vi "PH_PP_CurrentMeas_Stop.vi"(0 "connection ID in":refnum<k5>, 5 "error in (no error)":errorcluster) -> (14 "No Data achieved due to Task Failure":bool, 15 "Error unpacking Data?":bool, 16 "Measurement Data":waveform(dbl)[](graph), 17 "Receveived Data Sets":T1[](array[typedef]), 18 "No Data achieved due to no Trigger Signal":bool, 19 "error out":errorcluster)   [LabVIEW 2014, in "PH_PP_CurrentMeas.lvlib"]
uses:
  PH_PP_CurrentMeas.lvlib
  PH_PP_CurrentMeas.Command.ctl
  PH_PP_CurrentMeas.CommandCluster.ctl
panel:
  in  "Dummy":T1
  in  "Command":T2=enum."CloseConnection"
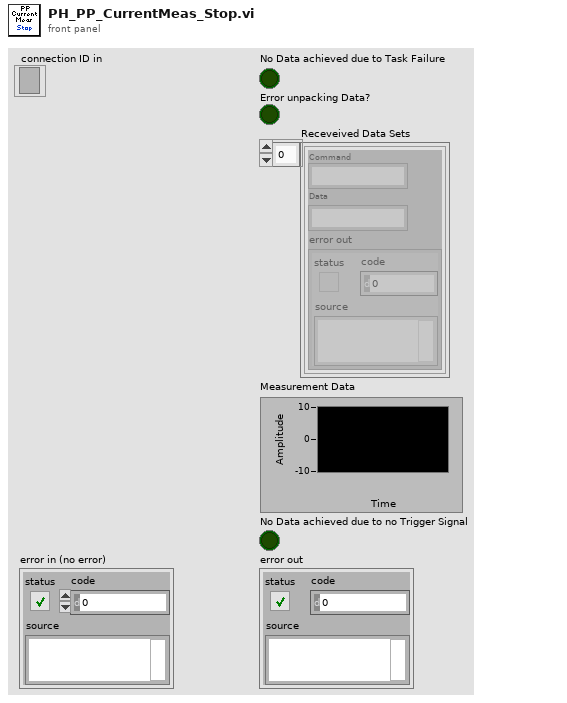
[diagram p1: front panel]
types:
  T1 = typedef "PH_PP_CurrentMeas.lvlib/PH_PP_CurrentMeas.CommandCluster.ctl" = cluster{"Command":string, "Data":string, "error out":errorcluster}
  T2 = typedef "PH_PP_CurrentMeas.lvlib/PH_PP_CurrentMeas.Command.ctl" = enum16{"StartDAQ", "StopDAQ", "GetDAQStatus", "CloseConnection"}
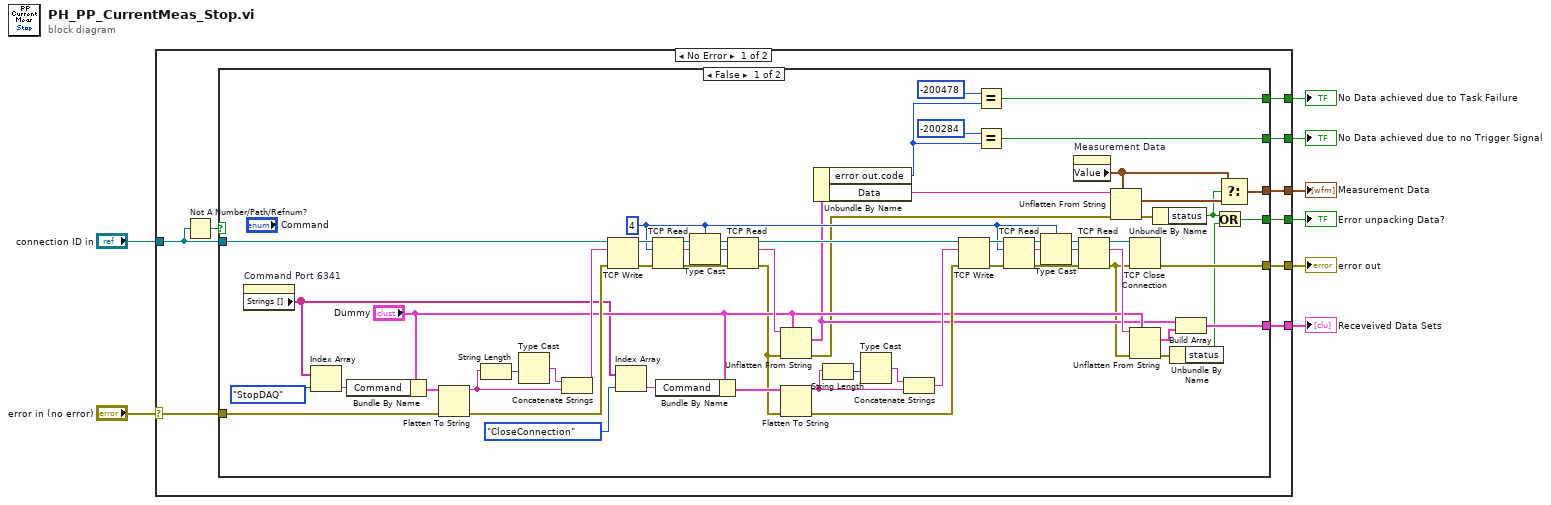
[diagram p0: block diagram]
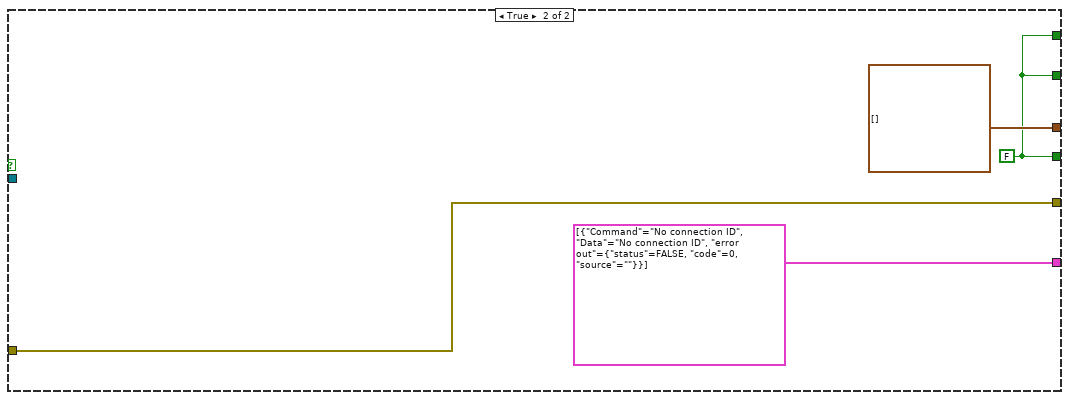
[diagram p2: hidden frame]
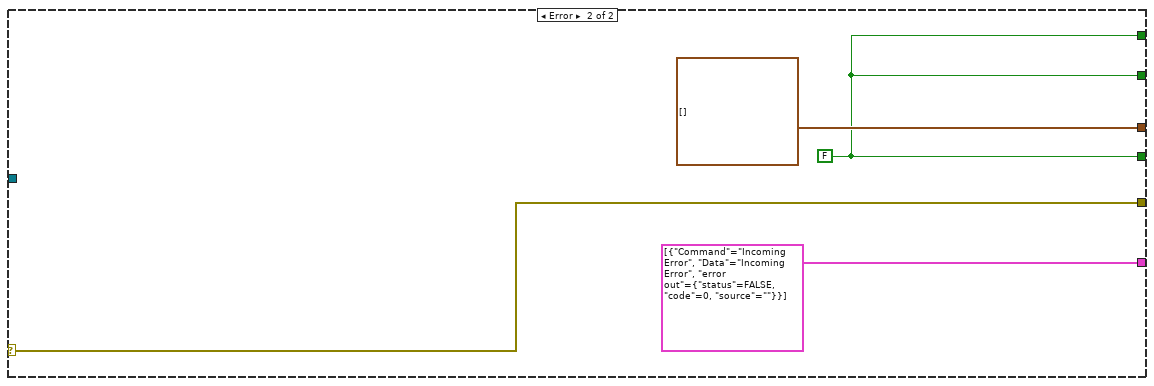
[diagram p3: hidden frame]
diagram:
  n1 = case shown="No Error" "error in (no error)" {
    selector: "error in (no error)" -> [w11 w83]
    tunnel: [w17 waveform(dbl)[] [] ("Value")] -> w8
    tunnel: "connection ID in" -> [w16 _]
    tunnel: [w15 w83] -> w6
    tunnel: [w14 T1[] [{"Command"="Incoming Error", "Data"="Incoming Error", "error out"={"status"=FALSE, "code"=0, "source"=""}}]] -> w5
    tunnel: [w12 w80] -> w4
    tunnel: [w10 w80] -> w2
    tunnel: [w9 w80] -> w1
    frame No Error {
      n2 = Not A Number/Path/Refnum?(number/path/refnum=w16) -> (NaN/Path/Refnum?=w13:bool)
      n3 = case shown="False" w13 {
        tunnel: [w57 waveform(dbl)[] [] ("Value")] -> w17
        tunnel: w11 -> [w56 w79]
        tunnel: w16 -> [w55 _]
        tunnel: [w54 w79] -> w15
        tunnel: [w32 T1[] [{"Command"="No connection ID", "Data"="No connection ID", "error out"={"status"=FALSE, "code"=0, "source"=""}}]] -> w14
        tunnel: [w24 w76] -> w12
        tunnel: [w21 w76] -> w10
        tunnel: [w18 w76] -> w9
        frame False {
          w34 = 4 ("bytes to read")
          n4 = property on="Command Port 6341" class="Enum (strict)"() -> ("Strings []"=w37:string[])  [unwired: 2 in, 2 out]
          n5 = Index Array(array=w37, index=PH_PP_CurrentMeas.Command."StopDAQ" ("Command")) -> (element=w75:string)
          n6 = Bundle By Name(cluster="Dummy", "Command"=w75) -> (w70:T1)
          n7 = Flatten To String(anything=w70, error in (no error)=w56) -> (data string=w72:string, error out=w69:errorcluster)  [unwired: 2 in, 1 out]
          n8 = String Length(string=w72) -> (length=w73:i32)
          n9 = Type Cast(x=w73) -> (*(type *) &x=w74:string)  [unwired: 1 in]
          n10 = Concatenate Strings(w74, w72) -> (w71:string)
          n11 = TCP Write(connection ID=w55, data in=w71, error in (no error)=w69) -> (connection ID out=w62:refnum<k5>, error out=w63:errorcluster)  [unwired: 1 in, 1 out]
          n12 = Index Array(array=w37, index=PH_PP_CurrentMeas.Command."CloseConnection" ("Command")) -> (element=w53:string)
          n13 = TCP Read(connection ID=w62, bytes to read=w34, error in (no error)=w63) -> (connection ID out=w66:refnum<k5>, data out=w64:string, error out=w67:errorcluster)  [unwired: 2 in]
          n14 = Bundle By Name(cluster="Dummy", "Command"=w53) -> (w48:T1)
          n15 = Type Cast(type=w34, x=w64) -> (*(type *) &x=w65:i32)
          n16 = TCP Read(connection ID=w66, bytes to read=w65, error in (no error)=w67) -> (connection ID out=w36:refnum<k5>, data out=w68:string, error out=w31:errorcluster)  [unwired: 2 in]
          n17 = Unflatten From String(type="Dummy", binary string=w68, error in (no error)=w31) -> (value=w33:T1, error out=w30:errorcluster)  [unwired: 2 in, 1 out]
          n18 = Flatten To String(anything=w48, error in (no error)=w31) -> (data string=w50:string, error out=w47:errorcluster)  [unwired: 2 in, 1 out]
          n19 = Unbundle By Name(w33) -> ("error out.code"=w19:i32, "Data"=w60:string)
          n20 = String Length(string=w50) -> (length=w51:i32)
          n21 = Type Cast(x=w51) -> (*(type *) &x=w52:string)  [unwired: 1 in]
          n22 = Concatenate Strings(w52, w50) -> (w49:string)
          n23 = TCP Write(connection ID=w36, data in=w49, error in (no error)=w47) -> (connection ID out=w40:refnum<k5>, error out=w41:errorcluster)  [unwired: 1 in, 1 out]
          n24 = Equal?(x=-200478, y=w19) -> (x = y?=w21:bool)
          n25 = Equal?(x=-200284, y=w19) -> (x = y?=w18:bool)
          n26 = TCP Read(connection ID=w40, bytes to read=w34, error in (no error)=w41) -> (connection ID out=w44:refnum<k5>, data out=w42:string, error out=w45:errorcluster)  [unwired: 2 in]
          n27 = Type Cast(type=w34, x=w42) -> (*(type *) &x=w43:i32)
          n28 = property on="Measurement Data" class="WFGraph (strict)"() -> ("Value"=w23:waveform(dbl)[])  [unwired: 2 in, 2 out]
          n29 = TCP Read(connection ID=w44, bytes to read=w43, error in (no error)=w45) -> (connection ID out=w35:refnum<k5>, data out=w46:string, error out=w28:errorcluster)  [unwired: 2 in]
          n30 = Unflatten From String(type=w23, binary string=w60, error in (no error)=w30) -> (value=w59:waveform(dbl)[], error out=w58:errorcluster)  [unwired: 2 in, 1 out]
          n31 = TCP Close Connection(connection ID=w35, error in (no error)=w28) -> (error out=w54:errorcluster)  [unwired: 1 in, 1 out]
          n32 = Unflatten From String(type="Dummy", binary string=w46, error in (no error)=w28) -> (value=w29:T1, error out=w27:errorcluster)  [unwired: 2 in, 1 out]
          n33 = Unbundle By Name(w58) -> ("status"=w26:bool)
          n34 = Unbundle By Name(w27) -> ("status"=w25:bool)
          n35 = Build Array(w33, w29) -> (w32:T1[])
          n36 = Or(x=w26, y=w25) -> (x .or. y?=w24:bool)
          n37 = Select(t=w23, s=w26, f=w59) -> (s? t:f=w57:waveform(dbl)[])
        }
        frame True {
          w76 = FALSE
        }
      }
    }
    frame Error {
      w80 = FALSE
    }
  }
  "error out" <- w6
  "Measurement Data" <- w8
  "Receveived Data Sets" <- w5
  "Error unpacking Data?" <- w4
  "No Data achieved due to Task Failure" <- w2
  "No Data achieved due to no Trigger Signal" <- w1
